vi "init.vi"(7 "io_timeout":u16, 8 "error in":errorcluster, 9 "io_2V8":bool, 10 "Slave Address(7 bit)":u8, 11 "I2C Ref In":T1) -> (0 "error out":errorcluster, 1 "status":bool, 2 "stop_variable":u8, 3 "I2C Ref Out":T1)   [LabVIEW 2018]
uses:
  <vilib>/myRIO/Instrument Drivers/Onboard IO/I2C/typedefs/I2C Reference.ctl
  <vilib>/myRIO/Common/Instrument Driver Framework/Utilities/typedefs/myRIO Generic Hardware Reference.ctl
  <vilib>/myRIO/Common/Instrument Driver Framework/Utilities/typedefs/Hardware Version Enum.ctl
  <vilib>/myRIO/Common/Instrument Driver Framework/Utilities/typedefs/myRIO v1.0 Reference.ctl
  <vilib>/myRIO/Common/Instrument Driver Framework/Utilities/typedefs/Generic FPGA Reference.ctl
  <vilib>/myRIO/Common/Instrument Driver Framework/myRIO v1.0/I2C/typedefs/I2C Channels Enum.ctl
  <vilib>/myRIO/Instrument Drivers/Onboard IO/I2C/typedefs/I2C Configuration.ctl
  <vilib>/myRIO/Instrument Drivers/Onboard IO/I2C/typedefs/I2C Transfer Rate.ctl
  <vilib>/Utility/error.llb/Error Cluster From Error Code.vi
  <vilib>/myRIO/Common/Instrument Driver Framework/myRIO v1.0/I2C/vis/myRIO v1.0 Write I2C.vi
  <vilib>/myRIO/Common/Instrument Driver Framework/myRIO v1.0/I2C/vis/myRIO v1.0 Read I2C.vi
  <vilib>/myRIO/Instrument Drivers/Onboard IO/I2C/I2C.lvlib
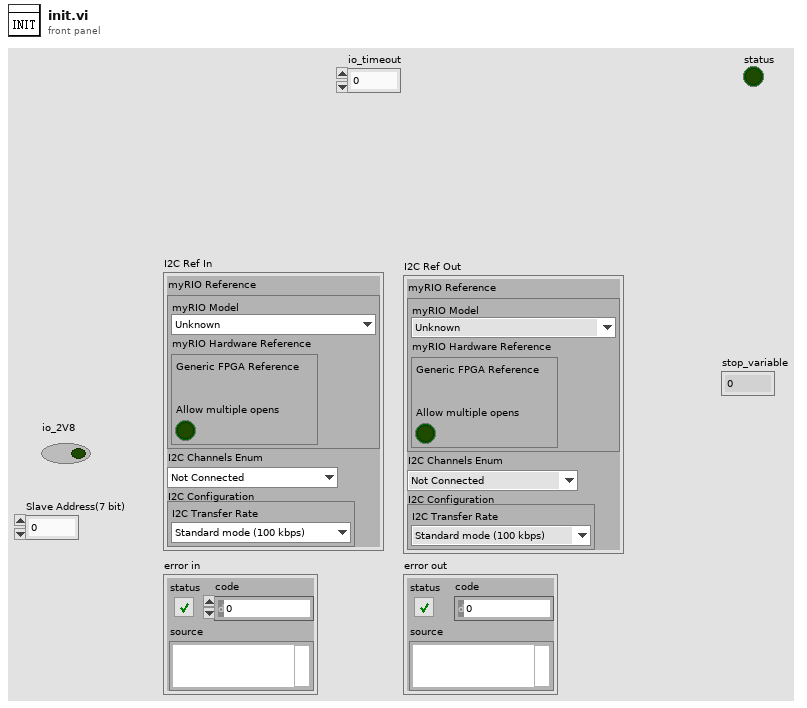
[diagram p1: front panel]
types:
  T1 = typedef "I2C.lvlib/I2C Reference.ctl" = cluster{"myRIO Reference":T2, "I2C Channels Enum":T6, "I2C Configuration":T7}
  T2 = typedef "myRIO Generic Hardware Reference.ctl" = cluster{"myRIO Model":T3, "myRIO Hardware Reference":T4}
  T3 = typedef "Hardware Version Enum.ctl" = enum16{"Unknown", "myRIO-1900", "myRIO-1950", "roboRIO", "NI ELVIS RIO CM", "ELVIS III"}
  T4 = typedef "myRIO v1.0 Reference.ctl" = cluster{"Generic FPGA Reference":T5, "Allow multiple opens":bool}
  T5 = typedef "Generic FPGA Reference.ctl" = refnum<k20>
  T6 = typedef "I2C Channels Enum.ctl" = enum16{"Not Connected", "A/I2C", "B/I2C", "I2C/I2C"}
  T7 = typedef "I2C.lvlib/I2C Configuration.ctl" = cluster{"I2C Transfer Rate":T8}
  T8 = typedef "I2C.lvlib/I2C Transfer Rate.ctl" = enum16{"Standard mode (100 kbps)", "Fast mode (400 kbps)"}
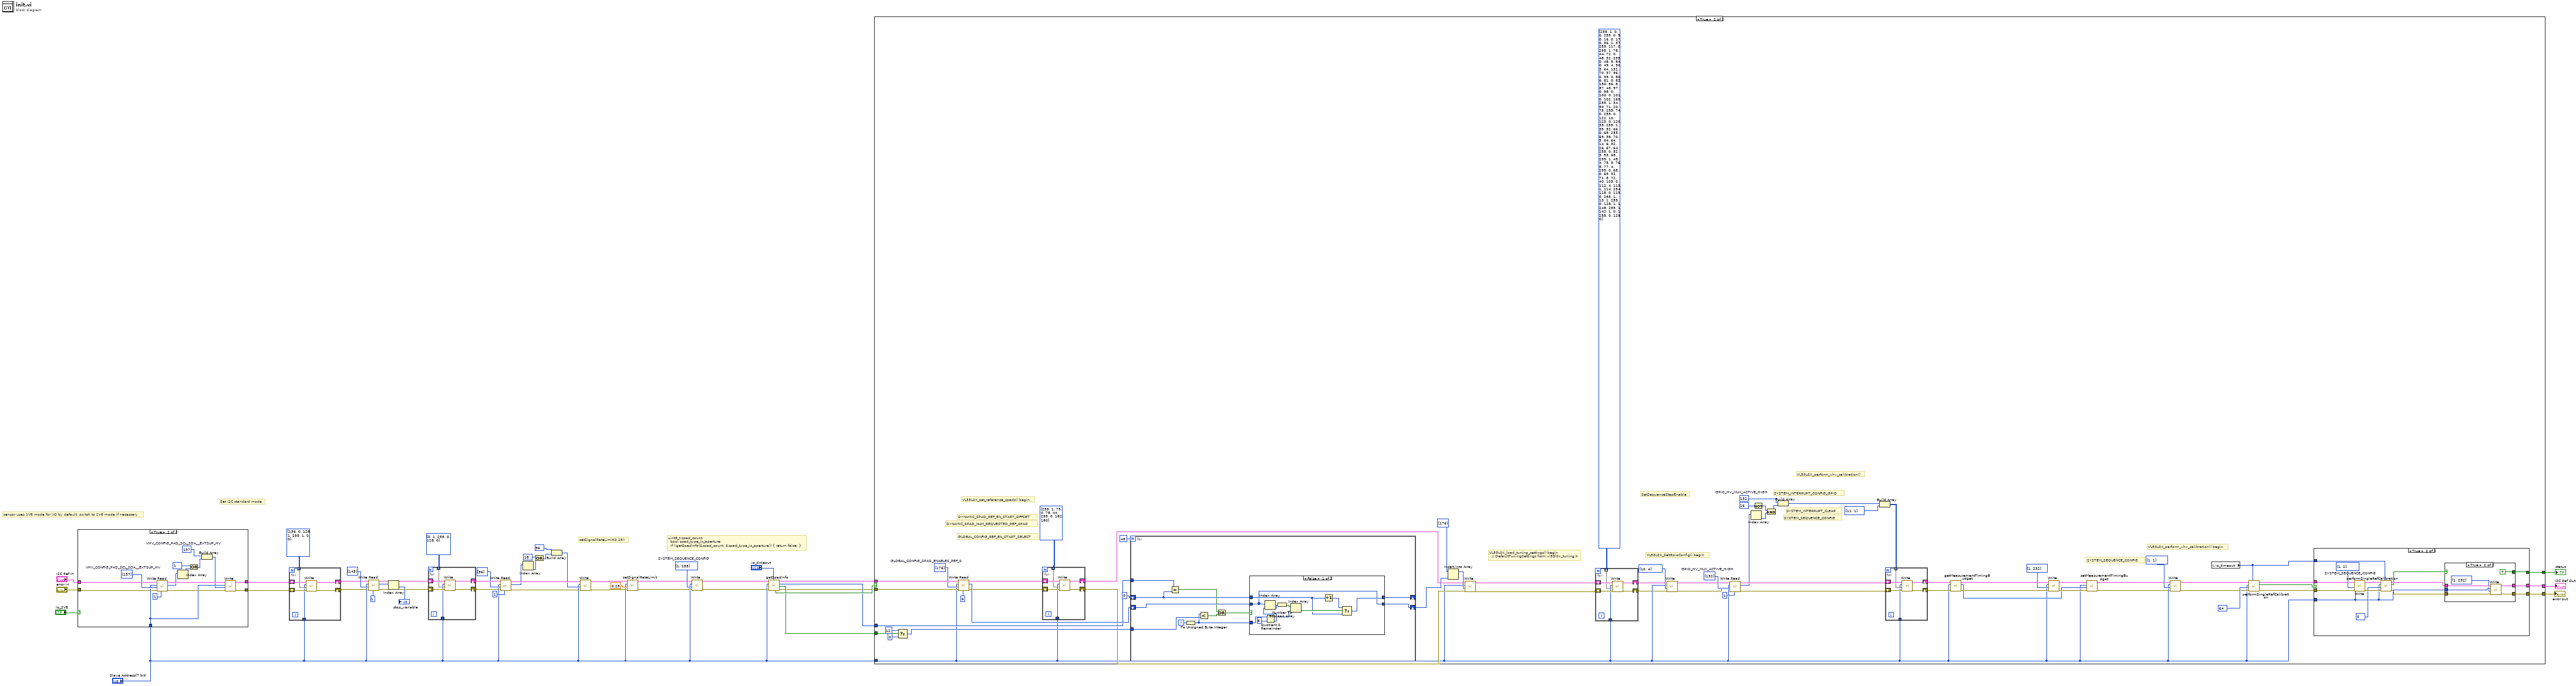
[diagram p0: block diagram]
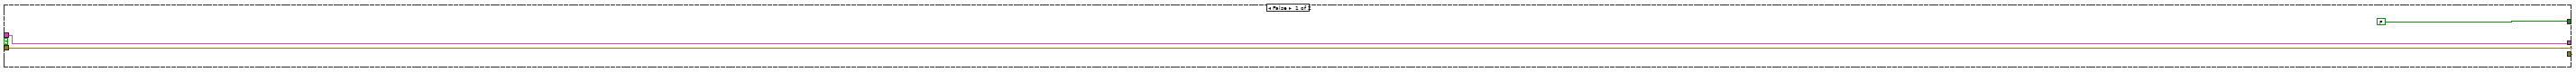
[diagram p2: hidden frame]
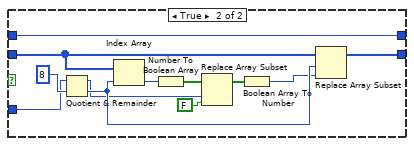
[diagram p5: hidden frame]
diagram:
  w28 = u8[] [1, 255]  # SYSTEM_SEQUENCE_CONFIG
  # "uint8_t spad_count;\n  bool spad_type_is_aperture;\n  if (!getSpadInfo(&spad_count, &spad_type_is_aperture)) { return false; }"
  # "setSignalRateLimit(0.25);"
  # "Set I2C standard mode"
  # "sensor uses 1V8 mode for I/O by default; switch to 2V8 mode if necessary"
  n1 = case shown="True" "io_2V8" {
    tunnel: [w47 w61] -> w41
    tunnel: [w46 w60] -> w9
    tunnel: "Slave Address(7 bit)" -> [_ w57]
    tunnel: "I2C Ref In" -> [w47 w56]
    tunnel: "error in" -> [w46 w55]
    frame False {
    }
    frame True {
      w49 = u8 137  # VHV_CONFIG_PAD_SCL_SDA__EXTSUP_HV
      w58 = u8[] [137]  # VHV_CONFIG_PAD_SCL_SDA__EXTSUP_HV
      n2 = call <vilib>:"Write Read.vi"("Byte Count"=u32 1, "error in (no error)"=w55, "Bytes to Write"=w58, "Slave Address (7-bit)"=w57, "I2C Ref In"=w56) -> ("error out"=w53:errorcluster, "Bytes Read"=w51:u8[], "I2C Ref Out"=w54:T1)  [unwired: 3 in]
      n3 = Index Array(array=w51) -> (element=w52:u8)  [unwired: 1 in]
      n4 = Or(x=u8 1, y=w52) -> (x .or. y?=w50:u8)
      n5 = Build Array(w49, w50) -> (w48:u8[])
      n6 = call <vilib>:"Write.vi"("error in (no error)"=w53, "Bytes to Write"=w48, "Slave Address (7-bit)"=w57, "I2C Ref In"=w54) -> ("error out"=w60:errorcluster, "I2C Ref Out"=w61:T1)  [unwired: 6 in]
    }
  }
  n7 = for {
    tunnel: u8[][] [[136, 0], [128, 1], [255, 1], [0, 0]] ("Bytes to Write") -> [w68] mode=indexing
    shift-right: [w64] -> w39
    shift-left: w41 -> [w67]
    shift-right: [w65] -> w10
    shift-left: w9 -> [w66]
    tunnel: "Slave Address(7 bit)" -> [w63]
    n8 = call <vilib>:"Write.vi"("error in (no error)"=w66, "Bytes to Write"=w68, "Slave Address (7-bit)"=w63, "I2C Ref In"=w67) -> ("error out"=w65:errorcluster, "I2C Ref Out"=w64:T1)  [unwired: 6 in]
  }
  n9 = call <vilib>:"Write Read.vi"("Byte Count"=u32 1, "error in (no error)"=w10, "Bytes to Write"=u8[] [145], "Slave Address (7-bit)"="Slave Address(7 bit)", "I2C Ref In"=w39) -> ("error out"=w11:errorcluster, "Bytes Read"=w27:u8[], "I2C Ref Out"=w37:T1)  [unwired: 3 in]
  n10 = Index Array(array=w27) -> (element=→"stop_variable":u8)  [unwired: 1 in]
  n11 = for {
    shift-right: [w71] -> w35
    shift-left: w37 -> [w74]
    shift-right: [w72] -> w13
    shift-left: w11 -> [w73]
    tunnel: "Slave Address(7 bit)" -> [w70]
    tunnel: u8[][] [[0, 1], [255, 0], [128, 0]] ("Bytes to Write") -> [w69] mode=indexing
    n12 = call <vilib>:"Write.vi"("error in (no error)"=w73, "Bytes to Write"=w69, "Slave Address (7-bit)"=w70, "I2C Ref In"=w74) -> ("error out"=w72:errorcluster, "I2C Ref Out"=w71:T1)  [unwired: 6 in]
  }
  n13 = call <vilib>:"Write Read.vi"("Byte Count"=u32 1, "error in (no error)"=w13, "Bytes to Write"=u8[] [96], "Slave Address (7-bit)"="Slave Address(7 bit)", "I2C Ref In"=w35) -> ("error out"=w12:errorcluster, "Bytes Read"=w31:u8[], "I2C Ref Out"=w33:T1)  [unwired: 3 in]
  n14 = Index Array(array=w31) -> (element=w7:u8)  [unwired: 1 in]
  n15 = Or(x=u8 18, y=w7) -> (x .or. y?=w8:u8)
  n16 = Build Array(u8 96, w8) -> (w29:u8[])
  n17 = call <vilib>:"Write.vi"("error in (no error)"=w12, "Bytes to Write"=w29, "Slave Address (7-bit)"="Slave Address(7 bit)", "I2C Ref In"=w33) -> ("error out"=w14:errorcluster, "I2C Ref Out"=w24:T1)  [unwired: 6 in]
  n18 = call "setSignalRateLimit.vi"("error in"=w14, "limit_Mcps"=0.25, "Slave Address (7-bit)"="Slave Address(7 bit)", "I2C Ref In"=w24) -> ("error out"=w22:errorcluster, "I2C Ref Out"=w23:T1)  [unwired: 5 in, 1 out]
  n19 = call <vilib>:"Write.vi"("error in (no error)"=w22, "Bytes to Write"=w28, "Slave Address (7-bit)"="Slave Address(7 bit)", "I2C Ref In"=w23) -> ("error out"=w5:errorcluster, "I2C Ref Out"=w6:T1)  [unwired: 6 in]
  n20 = call "getSpadInfo.vi"("io_timeout"="io_timeout", "error in"=w5, "Slave Address (7-bit)"="Slave Address(7 bit)", "I2C Ref In"=w6) -> ("error out"=w3:errorcluster, "type_is_aperture"=w19:bool, "count"=w18:u8, "I2C Ref Out"=w4:T1, "status"=w20:bool)  [unwired: 3 in]
  n21 = case shown="True" w20 {
    tunnel: w4 -> [w77 w140]
    tunnel: w3 -> [w76 w99]
    tunnel: [w77 w79] -> w2
    tunnel: [w76 w78] -> w1
    tunnel: "Slave Address(7 bit)" -> [_ w86]
    tunnel: w19 -> [_ w123]
    tunnel: w18 -> [_ w117]
    tunnel: [FALSE w106] -> w15
    frame False {
    }
    frame True {
      w126 = u8 132  # GPIO_HV_MUX_ACTIVE_HIGH
      w134 = u8[] [132]  # GPIO_HV_MUX_ACTIVE_HIGH
      w138 = u8[] [176]  # GLOBAL_CONFIG_SPAD_ENABLES_REF_0
      # "SYSTEM_INTERRUPT_CONFIG_GPIO"
      # "SYSTEM_INTERRUPT_CLEAR"
      # "SYSTEM_SEQUENCE_CONFIG"
      # "VL53L0X_perform_vhv_calibration() begin"
      # "VL53L0X_perform_vhv_calibration()"
      # "SYSTEM_SEQUENCE_CONFIG"
      # "SetSequenceStepEnable"
      # "VL53L0X_SetGpioConfig() begin"
      # "VL53L0X_load_tuning_settings() begin\n  // DefaultTuningSettings from vl53l0x_tuning.h"
      # "GLOBAL_CONFIG_REF_EN_START_SELECT"
      # "DYNAMIC_SPAD_NUM_REQUESTED_REF_SPAD"
      # "DYNAMIC_SPAD_REF_EN_START_OFFSET"
      # "VL53L0X_set_reference_spads() begin"
      n22 = Select(t=u8 12, s=w123, f=u8 0) -> (s? t:f=w119:u8)
      n23 = call <vilib>:"Write Read.vi"("Byte Count"=u32 6, "error in (no error)"=w99, "Bytes to Write"=w138, "Slave Address (7-bit)"=w86, "I2C Ref In"=w140) -> ("error out"=w100:errorcluster, "Bytes Read"=w118:u8[], "I2C Ref Out"=w101:T1)  [unwired: 3 in]
      n24 = for {
        shift-right: [w216] -> w98
        shift-left: w101 -> [w219]
        shift-right: [w217] -> w97
        shift-left: w100 -> [w218]
        tunnel: w86 -> [w215]
        tunnel: u8[][] [[255, 1], [79, 0], [78, 44], [255, 0], [182, 180]] ("Bytes to Write") -> [w214] mode=indexing
        n25 = call <vilib>:"Write.vi"("error in (no error)"=w218, "Bytes to Write"=w214, "Slave Address (7-bit)"=w215, "I2C Ref In"=w219) -> ("error out"=w217:errorcluster, "I2C Ref Out"=w216:T1)  [unwired: 6 in]
      }
      n26 = for {
        N: 48 -> [_]
        tunnel: w119 -> [w189]
        shift-right: [w187] -> w103
        shift-left: w118 -> [w188]
        tunnel: w117 -> [w186]
        shift-right: [w184] -> _
        shift-left: u8 0 ("spads_enabled") -> [w185]
        i -> [w190]
        n27 = Equal?(x=w186, y=w185) -> (x = y?=w181:bool)
        n28 = To Unsigned Byte Integer(number=w190) -> (unsigned 8bit integer=w183:u8)
        n29 = Less?(x=w183, y=w189) -> (x < y?=w182:bool)
        n30 = Or(x=w181, y=w182) -> (x .or. y?=w180:bool)
        n31 = case shown="False" w180 {
          tunnel: w183 -> [w201 w212]
          tunnel: w188 -> [w191 w211]
          tunnel: [w191 w209] -> w187
          tunnel: [w192 w208] -> w184
          tunnel: w185 -> [w193 w208]
          frame False {
            n32 = Quotient & Remainder(x=w201, y=u8 8) -> (x-y*floor(x/y)=w196:u8, floor(x/y)=w199:u8)
            n33 = Index Array(array=w191, index=w199) -> (element=w198:u8)
            n34 = Number To Boolean Array(number=w198) -> (Boolean array=w197:bool[])
            n35 = Index Array(array=w197, index=w196) -> (element=w195:bool)
            n36 = Increment(x=w193) -> (x+1=w194:u8)
            n37 = Select(t=w194, s=w195, f=w193) -> (s? t:f=w192:u8)
          }
          frame True {
            n38 = Quotient & Remainder(x=w212, y=u8 8) -> (x-y*floor(x/y)=w205:u8, floor(x/y)=w210:u8)
            n39 = Index Array(array=w211, index=w210) -> (element=w207:u8)
            n40 = Number To Boolean Array(number=w207) -> (Boolean array=w206:bool[])
            n41 = Replace Array Subset(array=w206, new element=FALSE ("new element/subarray"), index=w205) -> (w203:bool[])
            n42 = Boolean Array To Number(Boolean array=w203) -> (number=w202:u8)
            n43 = Replace Array Subset(array=w211, new element=w202, index=w210) -> (w209:u8[])
          }
        }
      }
      n44 = Insert Into Array(array=i32[] [176], new element=w103) -> (w102:i32[])  [unwired: 1 in]
      n45 = call <vilib>:"Write.vi"("error in (no error)"=w97, "Bytes to Write"=w102, "Slave Address (7-bit)"=w86, "I2C Ref In"=w98) -> ("error out"=w95:errorcluster, "I2C Ref Out"=w96:T1)  [unwired: 6 in]
      n46 = for {
        shift-right: [w176] -> w85
        shift-left: w96 -> [w179]
        shift-right: [w177] -> w84
        shift-left: w95 -> [w178]
        tunnel: w86 -> [w175]
        tunnel: u8[][] [[255, 1], [0, 0], [255, 0], [9, 0], [16, 0], [17, 0], [36, 1], [37, 255], [117, 0], [255, 1], [78, 44], [72, 0], [48, 32], [255, 0], [48, 9], [84, 0], [49, 4], [50, 3], [64, 131], [70, 37], [96, 0], [39, 0], [80, 6], [81, 0], [82, 150], [86, 8], [87, 48], [97, 0], [98, 0], [100, 0], [101, 0], [102, 160], [255, 1], [34, 50], [71, 20], [73, 255], [74, 0], [255, 0], [122, 10], [123, 0], [120, 33], [255, 1], [35, 52], [66, 0], [68, 255], [69, 38], [70, 5], [64, 64], [14, 6], [32, 26], [67, 64], [255, 0], [52, 3], [53, 68], [255, 1], [49, 4], [75, 9], [76, 5], [77, 4], [255, 0], [68, 0], [69, 32], [71, 8], [72, 40], [103, 0], [112, 4], [113, 1], [114, 254], [118, 0], [119, 0], [255, 1], [13, 1], [255, 0], [128, 1], [1, 248], [255, 1], [142, 1], [0, 1], [255, 0], [128, 0]] ("Bytes to Write") -> [w174] mode=indexing
        n47 = call <vilib>:"Write.vi"("error in (no error)"=w178, "Bytes to Write"=w174, "Slave Address (7-bit)"=w175, "I2C Ref In"=w179) -> ("error out"=w177:errorcluster, "I2C Ref Out"=w176:T1)  [unwired: 6 in]
      }
      n48 = call <vilib>:"Write.vi"("error in (no error)"=w84, "Bytes to Write"=u8[] [10, 4], "Slave Address (7-bit)"=w86, "I2C Ref In"=w85) -> ("error out"=w82:errorcluster, "I2C Ref Out"=w83:T1)  [unwired: 6 in]
      n49 = call <vilib>:"Write Read.vi"("Byte Count"=u32 1, "error in (no error)"=w82, "Bytes to Write"=w134, "Slave Address (7-bit)"=w86, "I2C Ref In"=w83) -> ("error out"=w132:errorcluster, "Bytes Read"=w129:u8[], "I2C Ref Out"=w133:T1)  [unwired: 3 in]
      n50 = Index Array(array=w129) -> (element=w128:u8)  [unwired: 1 in]
      n51 = Not(x=u8 16) -> (.not. x?=w130:u8)
      n52 = And(x=w130, y=w128) -> (x .and. y?=w127:u8)
      n53 = Build Array(w126, w127) -> (w94:u8[])
      n54 = Build Array(w94, u8[] [11, 1] ("Bytes to Write")) -> (w92:u8[][])
      n55 = for {
        shift-right: [w170] -> w91
        shift-left: w133 -> [w173]
        shift-right: [w171] -> w90
        shift-left: w132 -> [w172]
        tunnel: w92 -> [w169] mode=indexing
        tunnel: w86 -> [w168]
        n56 = call <vilib>:"Write.vi"("error in (no error)"=w172, "Bytes to Write"=w169, "Slave Address (7-bit)"=w168, "I2C Ref In"=w173) -> ("error out"=w171:errorcluster, "I2C Ref Out"=w170:T1)  [unwired: 6 in]
      }
      n57 = call "getMeasurementTimingBudget.vi"("error in"=w90, "Slave Address (7-bit)"=w86, "I2C Ref In"=w91) -> ("error out"=w88:errorcluster, "budget_us"=w113:u32, "I2C Ref Out"=w89:T1)  [unwired: 6 in]
      n58 = call <vilib>:"Write.vi"("error in (no error)"=w88, "Bytes to Write"=u8[] [1, 232], "Slave Address (7-bit)"=w86, "I2C Ref In"=w89) -> ("error out"=w114:errorcluster, "I2C Ref Out"=w115:T1)  [unwired: 6 in]
      n59 = call "setMeasurementTimingBudget.vi"("error in"=w114, "budget_us"=w113, "Slave Address (7-bit)"=w86, "I2C Ref In"=w115) -> ("error out"=w80:errorcluster, "I2C Ref Out"=w81:T1)  [unwired: 5 in, 1 out]
      n60 = call <vilib>:"Write.vi"("error in (no error)"=w80, "Bytes to Write"=u8[] [1, 1], "Slave Address (7-bit)"=w86, "I2C Ref In"=w81) -> ("error out"=w110:errorcluster, "I2C Ref Out"=w111:T1)  [unwired: 6 in]
      n61 = local read "io_timeout"() -> (w105:u16)
      n62 = call "performSingleRefCalibration.vi"("io_timeout"=w105, "error in"=w110, "vhv_init_byte"=u8 64, "Slave Address (7-bit)"=w86, "I2C Ref In"=w111) -> ("error out"=w108:errorcluster, "status"=w107:bool, "I2C Ref Out"=w109:T1)  [unwired: 4 in]
      n63 = case shown="True" w107 {
        selector: w107 -> [w143 _]
        tunnel: [w143 w145] -> w106
        tunnel: w86 -> [_ w148]
        tunnel: w109 -> [w142 w156]
        tunnel: w108 -> [w141 w155]
        tunnel: [w142 w147] -> w79
        tunnel: [w141 w146] -> w78
        tunnel: w105 -> [_ w144]
        frame False {
        }
        frame True {
          w157 = u8[] [1, 2]  # SYSTEM_SEQUENCE_CONFIG
          n64 = call <vilib>:"Write.vi"("error in (no error)"=w155, "Bytes to Write"=w157, "Slave Address (7-bit)"=w148, "I2C Ref In"=w156) -> ("error out"=w153:errorcluster, "I2C Ref Out"=w154:T1)  [unwired: 6 in]
          n65 = call "performSingleRefCalibration.vi"("io_timeout"=w144, "error in"=w153, "vhv_init_byte"=u8 0, "Slave Address (7-bit)"=w148, "I2C Ref In"=w154) -> ("error out"=w150:errorcluster, "status"=w149:bool, "I2C Ref Out"=w151:T1)  [unwired: 4 in]
          n66 = case shown="True" w149 {
            selector: w149 -> [w158 _]
            tunnel: w151 -> [w160 w167]
            tunnel: w150 -> [w159 w166]
            tunnel: w148 -> [_ w165]
            tunnel: [w160 w163] -> w147
            tunnel: [w159 w162] -> w146
            tunnel: [w158 TRUE] -> w145
            frame False {
            }
            frame True {
              n67 = call <vilib>:"Write.vi"("error in (no error)"=w166, "Bytes to Write"=u8[] [1, 232], "Slave Address (7-bit)"=w165, "I2C Ref In"=w167) -> ("error out"=w162:errorcluster, "I2C Ref Out"=w163:T1)  [unwired: 6 in]
            }
          }
        }
      }
    }
  }
  "I2C Ref Out" <- w2
  "error out" <- w1
  "status" <- w15
